vi "Funnel_Set.vi"   [LabVIEW 2020]
uses:
  Control_States_Funnel.ctl
  Funnel_Cluster.ctl
  Globals/Funnel_global.vi
types:
  T1 = typedef "Control_States_Funnel.ctl" = enum16{"No_Op", "Manual_Op"}
  T2 = typedef "Funnel_Cluster.ctl" = cluster{"Control States":T1, "Throttle":dbl}
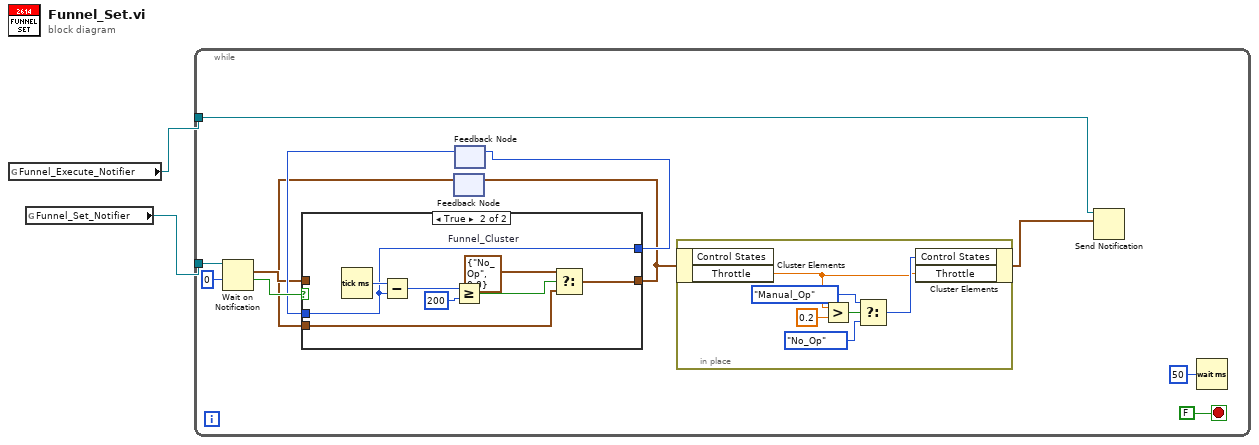
[diagram p0: block diagram]
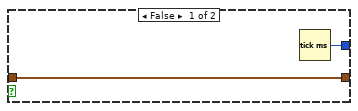
[diagram p2: hidden frame]
diagram:
  n1 = global read "Funnel_global.vi" "Funnel_Execute_Notifier"() -> (w2:refnum<notifier>)
  n2 = global read "Funnel_global.vi" "Funnel_Set_Notifier"() -> (w1:refnum<notifier>)
  n3 = while {
    tunnel: w1 -> [w6]
    tunnel: w2 -> [w3]
    stop <- FALSE stop-if-true
    n4 = Wait on Notification(notifier=w6, timeout in ms (-1)=0) -> (notification=w8:T2, timed out?=w11:bool)  [unwired: 2 in, 2 out]
    n5 = feedback #1() -> (w7:T2)  [unwired: 1 in]
    n6 = feedback #2() -> (w9:u32)  [unwired: 1 in]
    n7 = case shown="True" w11 {
      tunnel: w8 -> [w22 _]
      tunnel: [w22 w30] -> w5
      tunnel: w7 -> [_ w29]
      tunnel: [w21 w27] -> w10
      tunnel: w9 -> [_ w27]
      frame False {
        n8 = Tick Count (ms)() -> (millisecond timer value=w21:u32)
      }
      frame True {
        w23 = T2 {"Control States"=enum."No_Op", "Throttle"=0.0}  # Funnel_Cluster
        n9 = Tick Count (ms)() -> (millisecond timer value=w28:u32)
        n10 = Subtract(x=w28, y=w27) -> (x-y=w25:u32)
        n11 = Greater Or Equal?(x=w25, y=u32 200) -> (x >= y?=w26:bool)
        n12 = Select(t=w23, s=w26, f=w29) -> (s? t:f=w30:T2)
      }
    }
    n13 = feedback-in #1(w5) -> ()
    n14 = feedback-in #2(w10) -> ()
    n15 = in-place {
      n16 = in-place-cluster #3(w5) -> ("Throttle"=w15:dbl)  [unwired: 1 out]
      n17 = Greater?(x=w15, y=0.2) -> (0:w19:bool)
      n18 = Select(t=Control_States_Funnel."Manual_Op" ("Control States"), s=w19, f=Control_States_Funnel."No_Op" ("Control States")) -> (s? t:f=w16:T1)
      n19 = in-place-cluster #3("Control States"=w16, "Throttle"=w15) -> (w4:T2)
    }
    n20 = Send Notification(notification=w4, notifier=w3) -> ()  [unwired: 1 in, 2 out]
    n21 = Wait (ms)(milliseconds to wait=u32 50) -> ()  [unwired: 1 out]
  }
